vi "Log View for Band Power.vi"(3 "channel info":T1={"sensor sensitivity [mV/EU]"=1000.0, "engineering units"=1, "dB reference [EU]"=1.0, "custom label"="EU", "weighting filter"=0, "pregain [dB]"=0.0} {"pregain [dB]" format="%.2f"; "weighting filter" items=["Linear", "A-weighting", "B-weighting", "C-weighting", "ITU-R 468-4", "Dolby", "CCITT", "C-message"]; "dB reference [EU]" format="%^.1e"; "engineering units" items=["custom..."=0, "V"=1, "A"=21, "Pa"=2, "N"=20, "g"=3, "m/s^2"=4, "m/s"=5, "m"=6, "mm/s"=12, "mm"=13, "microns/s"=14, "microns"=15, "in/s^2"=7, "in/s"=8, "in"=9, "mils/s"=10, "mils"=11, "rad/s^2"=16, "rad/s"=17, "rad"=18, "strain"=19]; "sensor sensitivity [mV/EU]" format="%.2f"}, 4 "dB On (T)":bool=TRUE, 5 "band power [EU^2 rms]":dbl[](array[numeric]) format="%.2f") -> (0 "total band power [dB EU]":dbl format="%.2f", 1 "unit label":string, 2 "log view band power [dB EU]":dbl[](array[numeric]) format="%.2f")   [LabVIEW 2017]
uses:
  <vilib>/addons/Sound and Vibration/compatibility/Controls/svl_Channel Info.ctl
  <vilib>/addons/Sound and Vibration/compatibility/Controls/svl_Engineering Units Text Ring.ctl
  <vilib>/addons/Sound and Vibration/compatibility/Controls/svl_Weighting Filter Text Ring.ctl
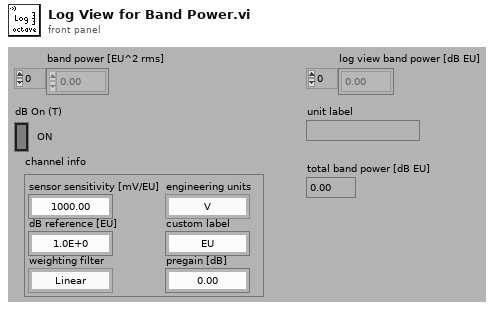
[diagram p1: front panel]
types:
  T1 = typedef "svl_Channel Info.ctl" = cluster{"sensor sensitivity [mV/EU]":dbl, "engineering units":T2, "dB reference [EU]":dbl, "custom label":string, "weighting filter":T3, "pregain [dB]":dbl}
  T2 = typedef "svl_Engineering Units Text Ring.ctl" = u16
  T3 = typedef "svl_Weighting Filter Text Ring.ctl" = u16
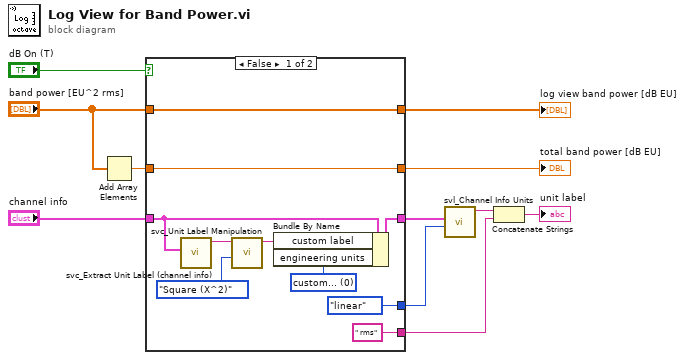
[diagram p0: block diagram]
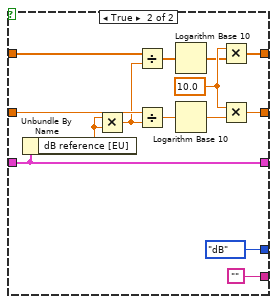
[diagram p2: hidden frame]
diagram:
  n1 = Add Array Elements(numeric array="band power [EU^2 rms]") -> (sum=w7:dbl)
  n2 = case shown="False" "dB On (T)" {
    tunnel: [w21 w35] -> w9
    tunnel: "channel info" -> [w13 w24]
    tunnel: "band power [EU^2 rms]" -> [w21 w34]
    tunnel: w7 -> [w20 w32]
    tunnel: [w20 w28] -> w6
    tunnel: [" rms" ""] -> w3
    tunnel: [enum16{"linear", "dB"}."linear" ("linear/dB") enum16{"linear", "dB"}."dB" ("linear/dB")] -> w2
    tunnel: [w12 w24] -> w1
    frame False {
      w16 = u16 0 items=["custom...", "V", "Pa", "g", "m/s^2", "m/s", "m", "in/s^2", "in/s", "in", "mm", "mils", "A"] ("engineering units")
      n3 = call <vilib>:"svc_Extract Unit Label (channel info).vi"("channel info"=w13) -> ("unit label"=w18:string)  [unwired: 8 in, 2 out]
      n4 = call <vilib>:"svc_Unit Label Manipulation.vi"("operation"=enum16{"Square (X^2)", "Divide (X/Y)"}."Square (X^2)", "X unit label"=w18) -> ("resulting unit label"=w17:string)  [unwired: 5 in]
      n5 = Bundle By Name(cluster=w13, "custom label"=w17, "engineering units"=w16) -> (w12:T1)
    }
    frame True {
      w26 = 10.0 ("y")
      n6 = Unbundle By Name(w24) -> ("dB reference [EU]"=w27:dbl)
      n7 = Multiply(x=w27, y=w27) -> (x*y=w31:dbl)
      n8 = Divide(x=w34, y=w31) -> (x/y=w33:dbl[])
      n9 = Divide(x=w32, y=w31) -> (x/y=w30:dbl)
      n10 = Logarithm Base 10(1:w33) -> (0:w25:dbl[])
      n11 = Logarithm Base 10(1:w30) -> (0:w29:dbl)
      n12 = Multiply(x=w26, y=w25) -> (x*y=w35:dbl[])
      n13 = Multiply(x=w26, y=w29) -> (x*y=w28:dbl)
    }
  }
  "log view band power [dB EU]" <- w9
  "total band power [dB EU]" <- w6
  n14 = call <vilib>:"svl_Channel Info Units.vi"("linear/dB"=w2, "channel info"=w1) -> ("unit label"=w5:string)  [unwired: 8 in, 1 out]
  n15 = Concatenate Strings(w5, w3) -> (→"unit label":string)
